vi "ZFFTunwrappedResult.vi"(6 "fft cluster acquisition":T1, 11 "result array out":dbl[][](array[numeric])) -> (1 "image":dbl[][](array[numeric]), 3 "modules FFT":dbl[][](array[numeric]))   [LabVIEW 2018]
uses:
  <vilib>/Analysis/2dsp.llb/Inverse Complex FFT.vi
  General Libraries/myFFT.lvlib
  <vilib>/Analysis/NI_AALPro.lvlib
panel:
  out "Intensity Graph":dbl[][](graph)
  in  "sequence NbX NbZ":dbl[][](array[numeric])
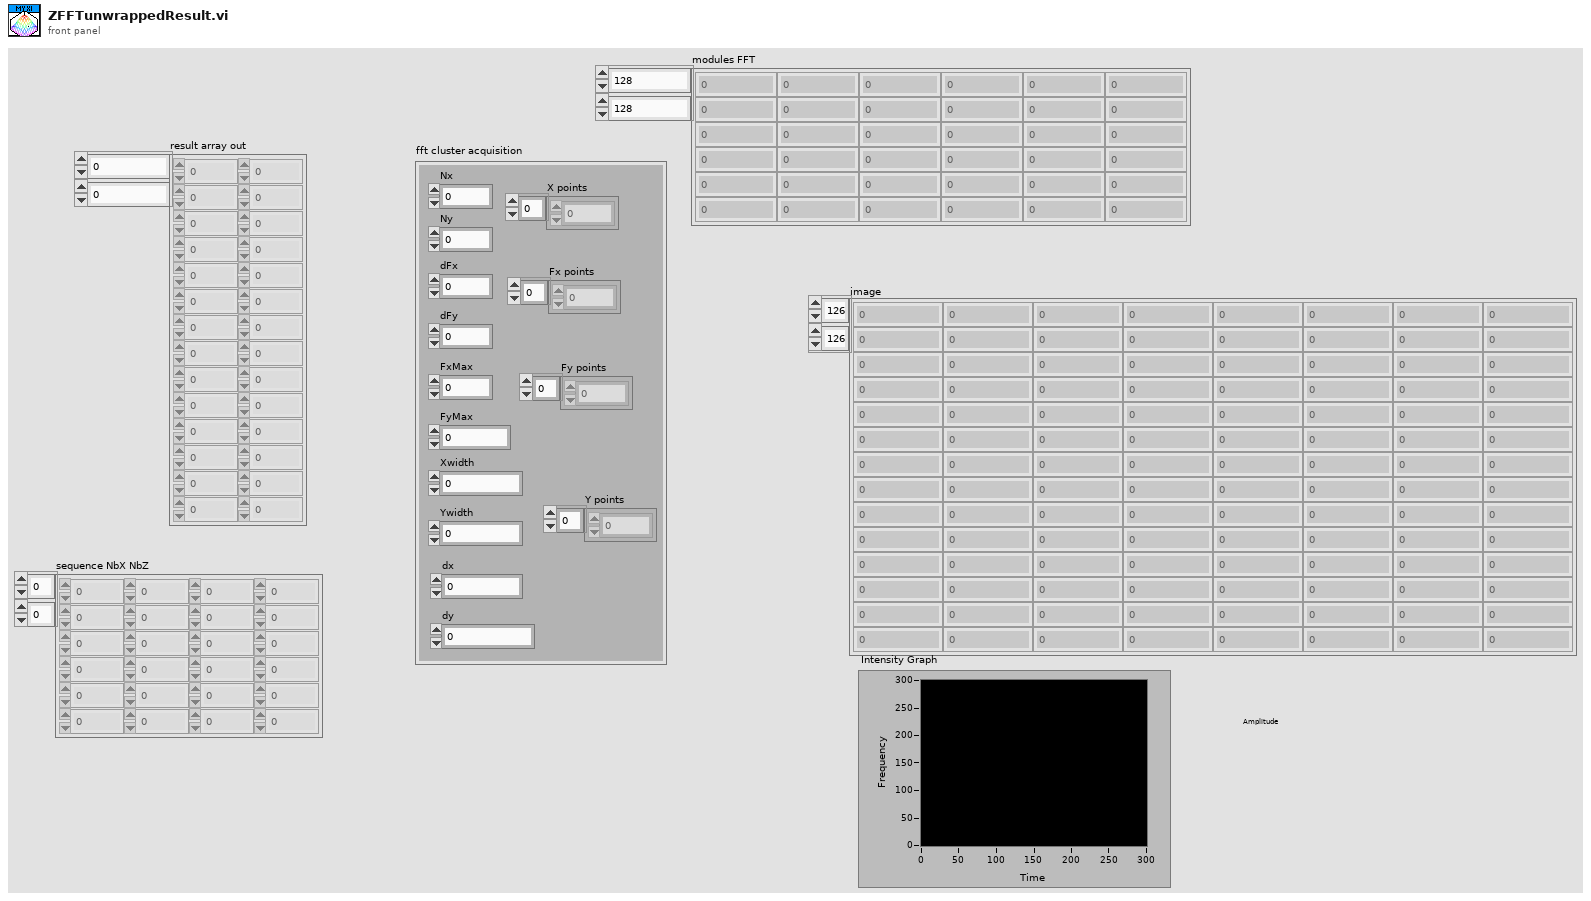
[diagram p1: front panel]
types:
  T1 = cluster{"dFx":dbl, "dFy":dbl, "Nx":i32, "Ny":i32, "FxMax":dbl, "FyMax":dbl, "Xwidth":dbl, "Ywidth":dbl, "dx":dbl, "dy":dbl, "Fx points":dbl[], "X points":dbl[], "Y points":dbl[], "Fy points":dbl[]}
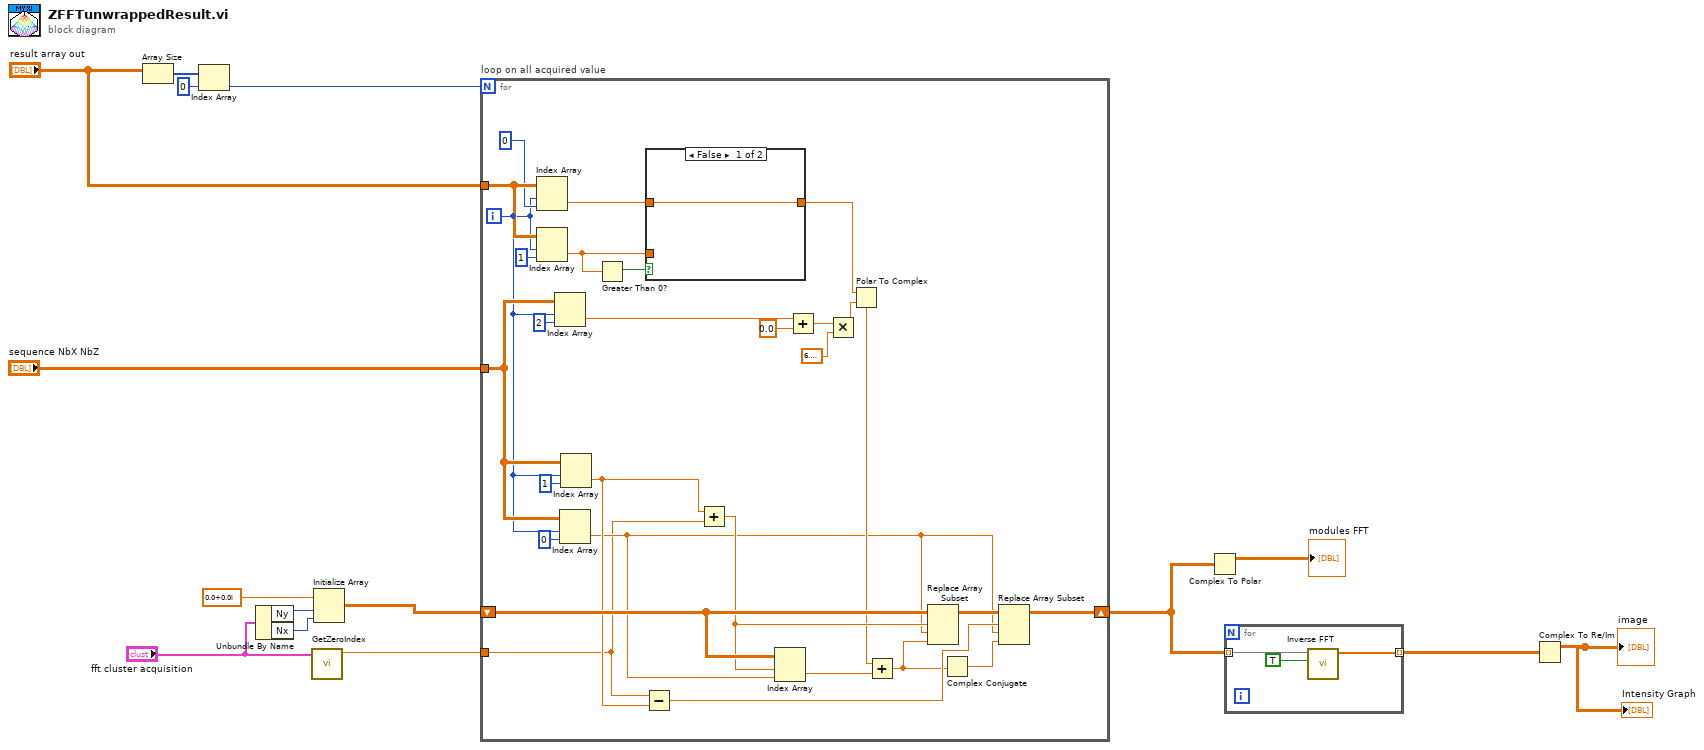
[diagram p0: block diagram]
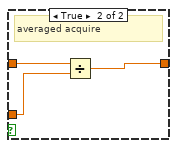
[diagram p2: hidden frame]
diagram:
  n1 = Array Size(array="result array out") -> (size(s)=w15:i32[])
  n2 = Index Array(array=w15, index=0) -> (element=w13:i32)
  n3 = Unbundle By Name("fft cluster acquisition") -> ("Ny"=w9:i32, "Nx"=w8:i32)
  n4 = call "GetZeroIndex.vi"("fft cluster"="fft cluster acquisition") -> ("Ny/2+1"=w1:dbl)  [unwired: 9 in, 1 out]
  n5 = Initialize Array(cdb 0.0+0.0i ("element"), w9, w8) -> (w7:cdb[][])
  n6 = for "loop on all acquired value" {
    N: w13 -> [_]
    tunnel: "sequence NbX NbZ" -> [w34]
    tunnel: "result array out" -> [w44]
    tunnel: w1 -> [w16]
    shift-right: [w24] -> w4
    shift-left: w7 -> [w30]
    i -> [w33]
    n7 = Index Array(array=w44, index (row)=w33, index (col)=0 ("disabled index (col)")) -> (element=w42:dbl)
    n8 = Index Array(array=w44, index (row)=w33, index (col)=1 ("disabled index (col)")) -> (element=w40:dbl)
    n9 = Index Array(array=w34, index (row)=w33, index (col)=2 ("disabled index (col)")) -> (element=w21:dbl)
    n10 = Index Array(array=w34, index (row)=w33, index (col)=0 ("disabled index (col)")) -> (element=w17:dbl)
    n11 = Index Array(array=w34, index (row)=w33, index (col)=1 ("disabled index (col)")) -> (element=w19:dbl)
    n12 = Greater Than 0?(x=w40) -> (x > 0?=w41:bool)
    n13 = Subtract(x=w16, y=w19) -> (x-y=w25:dbl)
    n14 = case shown="False" w41 {
      tunnel: w42 -> [w45 w48]
      tunnel: w40 -> [_ w47]
      tunnel: [w45 w46] -> w36
      frame False {
      }
      frame True {
        # "averaged acquire"
        n15 = Divide(x=w48, y=w47) -> (x/y=w46:dbl)
      }
    }
    n16 = Add(x=w19, y=w16) -> (x+y=w29:dbl)
    n17 = Index Array(array=w30, index (row)=w29, index (col)=w17) -> (element=w28:cdb)
    n18 = Add(x=w21, y=0.0) -> (x+y=w20:dbl)
    n19 = Multiply(x=w20, y=6.283185307179586) -> (x*y=w35:dbl)
    n20 = Polar To Complex(1:w35, 2:w36) -> (0:w27:cdb)
    n21 = Add(x=w27, y=w28) -> (x+y=w23:cdb)
    n22 = Replace Array Subset(array=w30, new element=w23, index (row)=w29, index (col)=w17) -> (w26:cdb[][])
    n23 = Complex Conjugate(1:w23) -> (0:w22:cdb)
    n24 = Replace Array Subset(array=w26, new element=w22, index (row)=w25, index (col)=w17) -> (w24:cdb[][])
  }
  n25 = Complex To Polar(r * e^(i*theta)=w4) -> (r=→"modules FFT":dbl[][])  [unwired: 1 out]
  n26 = for {
    tunnel: w4 -> [w50] mode=indexing
    tunnel: [w49] -> w3 mode=indexing
    n27 = call-poly <vilib>:"Inverse FFT.vi"("shift?"=TRUE, "FFT {X}"=w50) -> ("X"=w49:cdb[])  [unwired: 8 in, 1 out]
  }
  n28 = Complex To Re/Im(x + iy=w3) -> (x=→"image" →"Intensity Graph":dbl[][])  [unwired: 1 out]
